vi "Stop a Motor.vi"(8 "error in (no error)":errorcluster, 10 "index":i32, 11 "Motions in":refnum<class "Motions.lvclass">) -> (0 "error out":errorcluster, 3 "Motions out":refnum<class "Motions.lvclass">)   [LabVIEW 2016, in "Hardware.lvlib" / "Motions.lvlib" / "Motions.lvclass"]
uses:
  <userlib>/Common Components/Hardware/Abstract System/Motions/Motions/Motions.lvclass
  <userlib>/Common Components/Hardware/Abstract System/Motions/Motions/Motions.lvclass/Motions.ctl
  <userlib>/Common Components/Hardware/Motor/Motor/Motor.lvclass
  <userlib>/Common Components/TriggerAction Q/TriggerAction Q/TriggerAction Q.lvclass
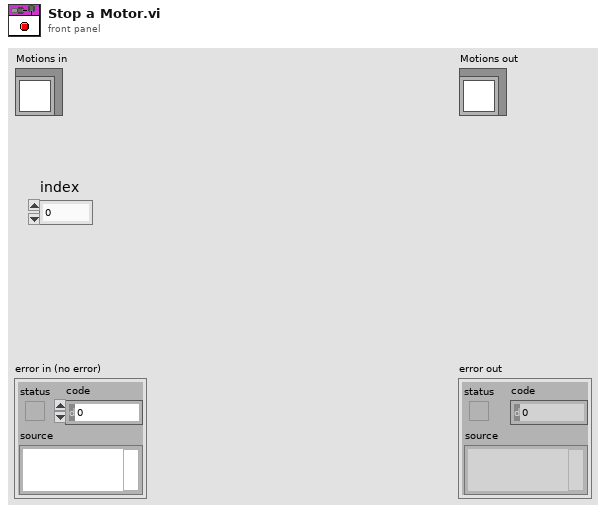
[diagram p1: front panel]
types:
  T1 = typedef "Hardware.lvlib/Motions.lvlib/Motions.lvclass/Motor States.ctl" = cluster{"Connected":bool, "Enabled":bool, "Moving Status":bool, "Soft Moving Status":bool, "Current Pos":dbl, "Target Pos":dbl, "Moving Dir (-1, 0, 1)":i32, "Error Status":bool, "Hard Limit+":bool, "Hard Limit-":bool, "Soft Limit+":bool, "Soft Limit-":bool, "History Dst Stack":refnum<queue>, "Motion Status":bool, "Motion TriggerAction Obj":refnum<class "TriggerAction Q.lvclass">}
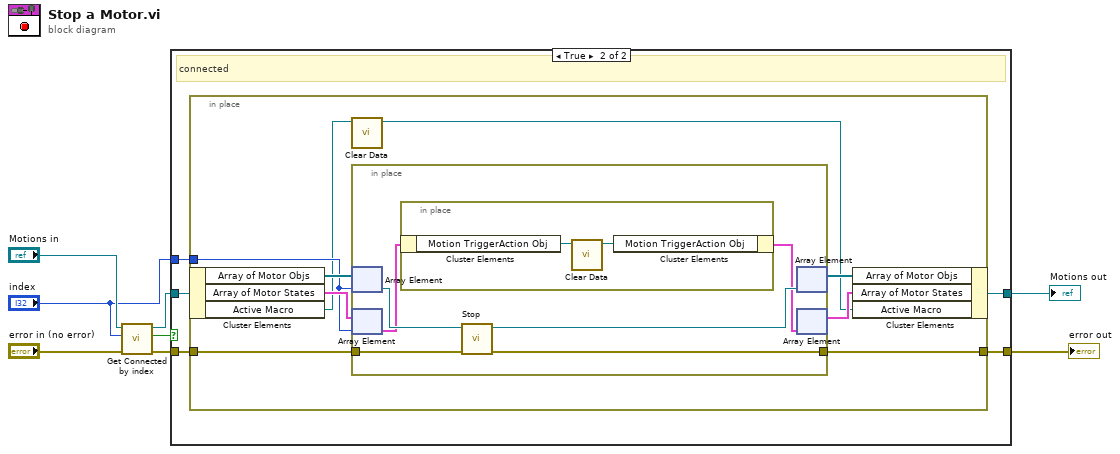
[diagram p0: block diagram]
diagram:
  n1 = call <userlib>:"Get Connected by index.vi"("error in (no error)"="error in (no error)", "index"="index", "Motions in"="Motions in") -> ("error out"=w5:errorcluster, "Connected"=w1:bool, "Motions out"=w3:refnum<class "Motions.lvclass">)  [unwired: 6 in]
  n2 = case shown="True" w1 {
    tunnel: [w9 w15] -> w8
    tunnel: [w10 w14] -> w6
    tunnel: w5 -> [w10 w13]
    tunnel: w3 -> [w9 w11]
    tunnel: "index" -> [_ w12]
    frame False {
    }
    frame True {
      # "connected"
      n3 = in-place {
        in-place-border: w12 -> [w18]
        in-place-border: w13 -> [w22]
        in-place-border: [w21] -> w14
        n4 = in-place-cluster #1(w11) -> ("Array of Motor Objs"=w24:refnum<class "Motor.lvclass">[], "Array of Motor States"=w20:T1[], "Active Macro"=w17:refnum<class "TriggerAction Q.lvclass">)
        n5 = call <userlib>:"Clear Data.vi"("TriggerAction in"=w17) -> ("TriggerAction out"=w16:refnum<class "TriggerAction Q.lvclass">)  [unwired: 9 in, 1 out]
        n6 = in-place {
          in-place-border: w22 -> [w28]
          in-place-border: [w27] -> w21
          n7 = in-place-array #2(w24, w18) -> (w30:refnum<class "Motor.lvclass">)
          n8 = in-place-array #3(w20, w18) -> (w26:T1)
          n9 = in-place {
            n10 = in-place-cluster #4(w26) -> ("Motion TriggerAction Obj"=w31:refnum<class "TriggerAction Q.lvclass">)
            n11 = call <userlib>:"Clear Data.vi"("TriggerAction in"=w31) -> ("TriggerAction out"=w32:refnum<class "TriggerAction Q.lvclass">)  [unwired: 9 in, 1 out]
            n12 = in-place-cluster #4("Motion TriggerAction Obj"=w32) -> (w25:T1)
          }
          n13 = call-dynamic "Stop.vi"("error in (no error)"=w28, "Motor in"=w30) -> ("error out"=w27:errorcluster, "Motor out"=w29:refnum<class "Motor.lvclass">)  [unwired: 8 in]
          n14 = in-place-array #2(w29) -> (w23:refnum<class "Motor.lvclass">[])  [unwired: 1 out]
          n15 = in-place-array #3(w25) -> (w19:T1[])  [unwired: 1 out]
        }
        n16 = in-place-cluster #1("Array of Motor Objs"=w23, "Array of Motor States"=w19, "Active Macro"=w16) -> (w15:refnum<class "Motions.lvclass">)
      }
    }
  }
  "error out" <- w6
  "Motions out" <- w8
